vi "test.vi"() -> ()   [LabVIEW 2020]
uses:
  <instrlib>/Agilent ENA Series/Agilent ENA Series.lvlib
panel:
  out "XY Graph":T1(graph)
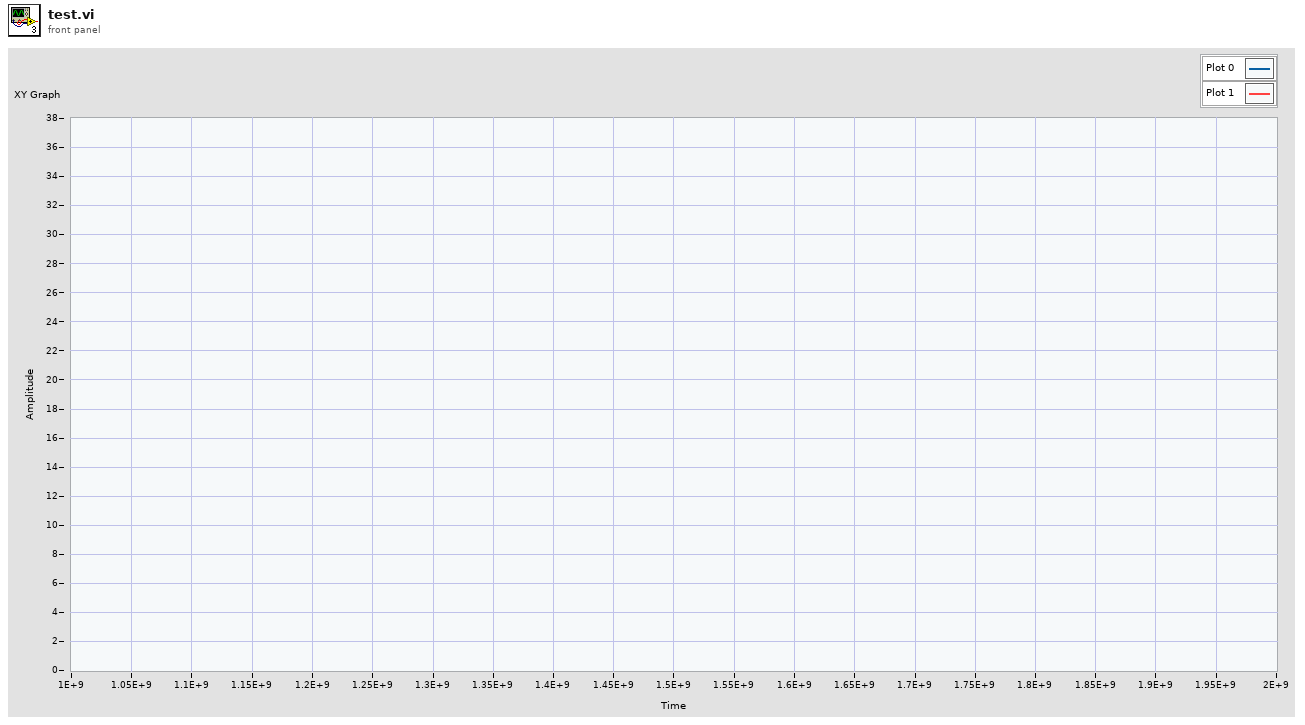
[diagram p1: front panel]
types:
  T1 = cluster{"Start Point X Value (0.0)":dbl[], dbl[]}[]
  T2 = cluster{"Start Point X Value (0.0)":dbl[], dbl[]}
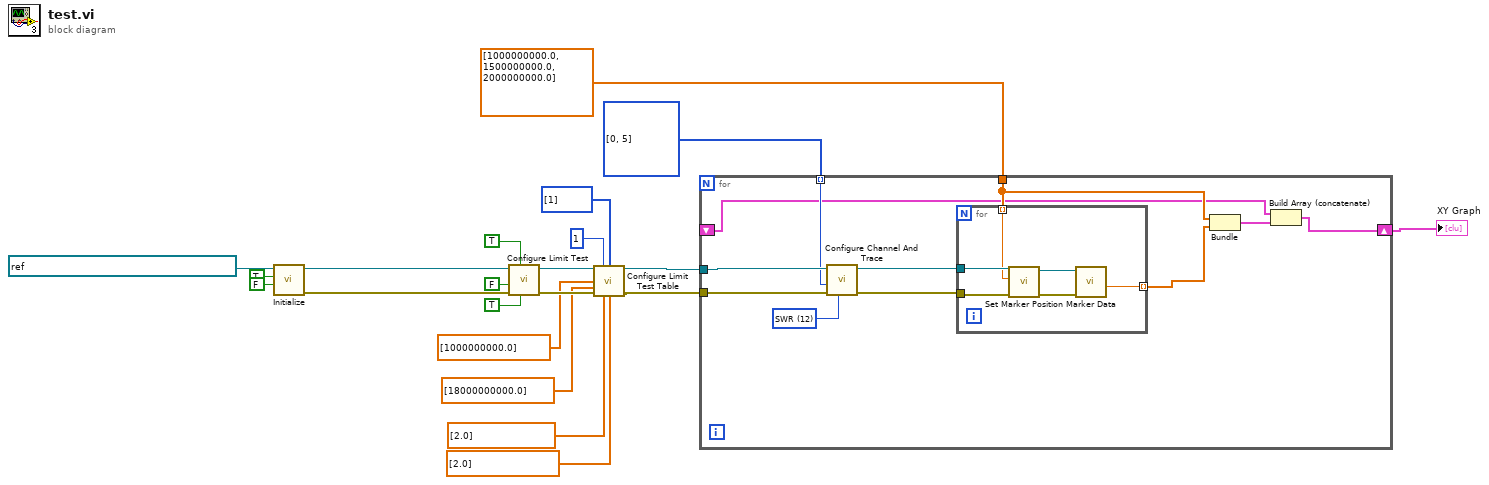
[diagram p0: block diagram]
diagram:
  w2 = u16[] [0, 5] items=["S11", "S21", "S31", "S41", "S12", "S22", "S32", "S42", "S13", "S23", "S33", "S43", "S14", "S24", "S34", "S44", "A", "B", "C", "D", "R1", "R2", "R3", "R4", "AUX1", "AUX2", "TR", "T", "R"]
  n1 = call <instrlib>:"Initialize.vi"("Reset? (T: Yes)"=FALSE, "ID Query? (T: Yes)"=TRUE, "VISA resource name"=refnum<visa-resource-name> "TCPIP0::192.168.1.111::inst0::INSTR") -> ("error out"=w5:errorcluster, "VISA resource name out"=w6:refnum<visa-resource-name>)  [unwired: 7 in]
  n2 = call <instrlib>:"Configure Limit Test.vi"("Limit Line Display (F: Disable)"=TRUE, "Limit Test (F: Disable)"=TRUE, "error in (no error)"=w5, "Limit Fail Display (F: Disable)"=FALSE, "VISA resource name"=w6) -> ("error out"=w18:errorcluster, "VISA resource name out"=w19:refnum<visa-resource-name>)  [unwired: 5 in]
  n3 = call <instrlib>:"Configure Limit Test Table.vi"("VISA resource name"=w19, "Number of Lines (0)"=1, "Type of Line (0)"=i32[] [1], "Start Point X Value (0.0)"=dbl[] [1000000000.0], "End Point X Value (0.0)"=dbl[] [18000000000.0] ("Start Point X Value (0.0)"), "error in (no error)"=w18, "Start Point Y Value (0.0)"=dbl[] [2.0] ("Start Point X Value (0.0)"), "End Point Y Value (0.0)"=dbl[] [2.0] ("Start Point X Value (0.0)")) -> ("VISA resource name out"=w3:refnum<visa-resource-name>, "error out"=w4:errorcluster)  [unwired: 6 in]
  n4 = for {
    tunnel: dbl[] [1000000000.0, 1500000000.0, 2000000000.0] ("Start Point X Value (0.0)") -> [w26]
    tunnel: w4 -> [w31]
    tunnel: w3 -> [w30]
    tunnel: w2 -> [w27] mode=indexing
    shift-right: [w22] -> w1
    shift-left: _ -> [w23]
    w32 = u16 12 items=["Logarithmic Magnitude", "Phase", "Group Delay", "Smith Chart  Linear (Lin/Phase)", "Smith Chart  Logarithmic (Log/Phase)", "Smith Chart  Complex (Real/Imag)", "Smith Chart  Impedance (R+jX)", "Smith Chart  Admittance (G+jB)", "Polar Format (Linear)", "Polar Format (Logarithmic)", "Polar Format (Re/Im)", "Linear Magnitude", "SWR", "Real", "Imaginary", "Epanded Phase", "Positive Phase"] ("Data Format (0: Logarithmic Magnitude)")
    n5 = call <instrlib>:"Configure Channel And Trace.vi"("Data Format (0: Logarithmic Magnitude)"=w32, "error in (no error)"=w31, "Measurement Parameters (0: S11)"=w27, "VISA resource name"=w30) -> ("error out"=w28:errorcluster, "VISA resource name out"=w29:refnum<visa-resource-name>)  [unwired: 6 in]
    n6 = for {
      tunnel: w28 -> [w36]
      tunnel: w29 -> [w35]
      tunnel: w26 -> [w34] mode=indexing
      tunnel: [w33] -> w25 mode=indexing
      n7 = call <instrlib>:"Set Marker Position.vi"("error in (no error)"=w36, "X Value (0.0)"=w34, "VISA resource name"=w35) -> ("error out"=w37:errorcluster, "VISA resource name out"=w38:refnum<visa-resource-name>)  [unwired: 7 in]
      n8 = call <instrlib>:"Marker Data.vi"("error in (no error)"=w37, "VISA resource name"=w38) -> ("Y Real Value"=w33:dbl)  [unwired: 5 in, 4 out]
    }
    n9 = Bundle("Start Point X Value (0.0)"=w26, w25) -> (w24:T2)  [unwired: 1 in]
    n10 = Build Array (concatenate)(w23, w24) -> (w22:T1)
  }
  "XY Graph" <- w1
